vi "AlliGator Save FLI Dataset Metadata.vi"(6 "Dataset Timestamp":dbl, 7 "Gate Image File Name":string, 8 "error in":errorcluster, 9 "Metadata":string, 10 "DAQ Parameters":T1, 11 "selected path":path) -> (0 "error out":errorcluster, 1 "Message":string, 3 "Saved Metadata File Path":path)   [LabVIEW 2021, in "AlliGator Files.lvlib"]
uses:
  AlliGator Files.lvlib
  Phasor/Phasor Fluorescence Lifetime Parameters v3.ctl
  Variant/Variant.lvlib
  Phasor/Phasor.lvlib
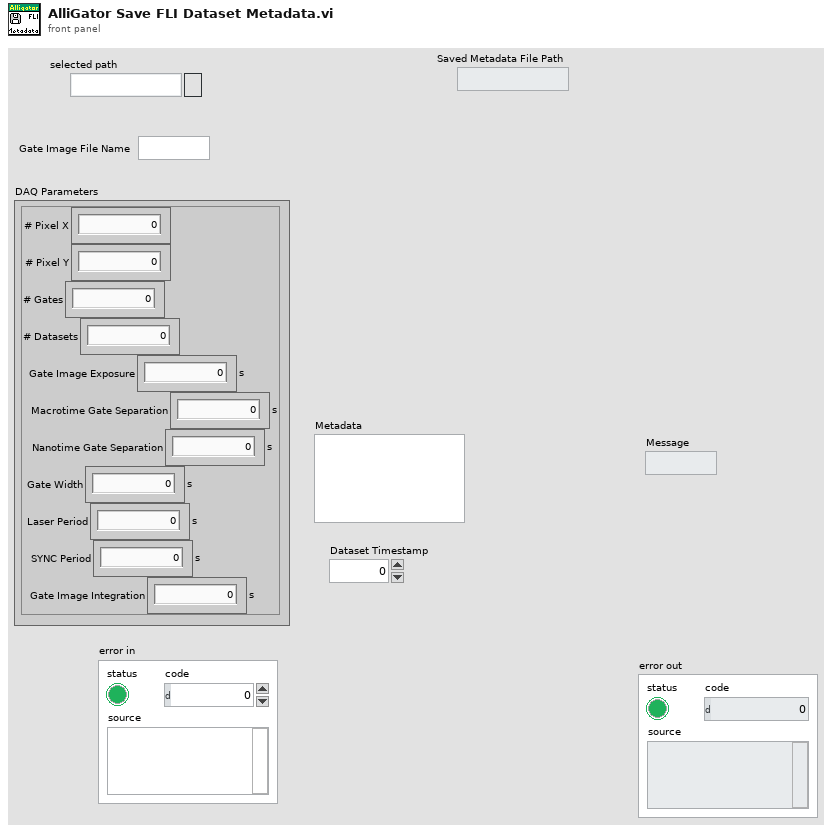
[diagram p1: front panel]
types:
  T1 = typedef "Phasor.lvlib/Phasor Fluorescence Lifetime Parameters v3.ctl" = cluster{"# Pixel X":i32, "# Pixel Y":i32, "# Gates":i32, "# Datasets":i32, "Gate Image Exposure":dbl[unit], "Macrotime Gate Separation":dbl[unit], "Nanotime Gate Separation":dbl[unit], "Gate Width":dbl[unit], "Laser Period":dbl[unit], "SYNC Period":dbl[unit], "Gate Image Integration":dbl[unit]}
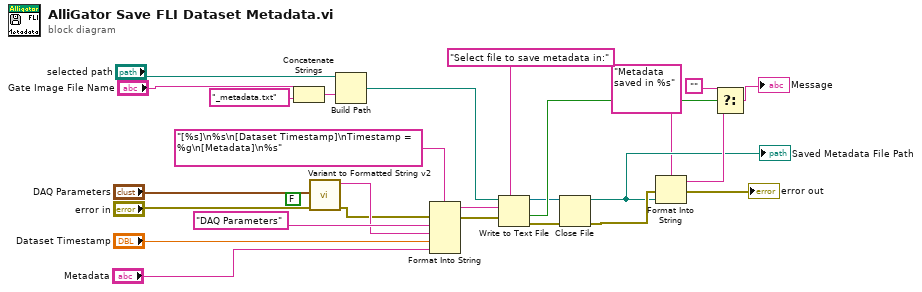
[diagram p0: block diagram]
diagram:
  (unwired) FALSE ("Hide Long Cluster Names (T)")
  n1 = Concatenate Strings("Gate Image File Name", "_metadata.txt" ("string")) -> (w6:string)
  n2 = call "Variant to Formatted String v2.vi"("error in (no error)"="error in", "Anything"="DAQ Parameters") -> ("error out"=w11:errorcluster, "String"=w12:string)  [unwired: 8 in]
  n3 = Build Path(base path="selected path", name or relative path=w6) -> (appended path=w5:path)
  n4 = Format Into String(format string="[%s]\n%s\n[Dataset Timestamp]\nTimestamp = %g\n[Metadata]\n%s", error in=w11, "DAQ Parameters" ("Label"), w12, "Dataset Timestamp", "Metadata") -> (resulting string=w9:string, error out=w8:errorcluster)  [unwired: 1 in]
  n5 = Write to Text File(prompt (Choose or enter file path)="Select file to save metadata in:", file (use dialog)=w5, text=w9, error in=w8) -> (refnum out=w3:refnum<file>, cancelled=w21:bool, error out=w2:errorcluster)
  n6 = Close File(refnum=w3, error in=w2) -> (path=w19:path, error out=w20:errorcluster)
  "Saved Metadata File Path" <- w19
  n7 = Format Into String(format string="Metadata saved in %s", error in=w20, w19) -> (resulting string=w22:string, error out=→"error out":errorcluster)  [unwired: 1 in]
  n8 = Select(t="", s=w21, f=w22) -> (s? t:f=→"Message":string)
